vi "Read Shake Data.vi"(8 "error in (no error)":errorcluster, 11 "Abstract Shake Monitor in":refnum<class "Abstract Shake Monitor.lvclass">) -> (0 "error out":errorcluster, 1 "Shake Amplitude (g)":dbl, 2 "Shake Frequency (Hz)":dbl, 3 "Abstract Shake Monitor out":refnum<class "Abstract Shake Monitor.lvclass">)   [LabVIEW 2020, in "Shaker Controller.lvlib" / "Abstract Shake Monitor.lvclass"]
uses:
  Abstract Shake Monitor.lvclass
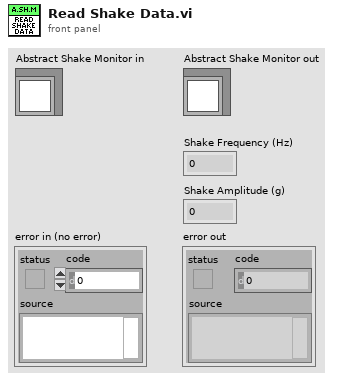
[diagram p1: front panel]
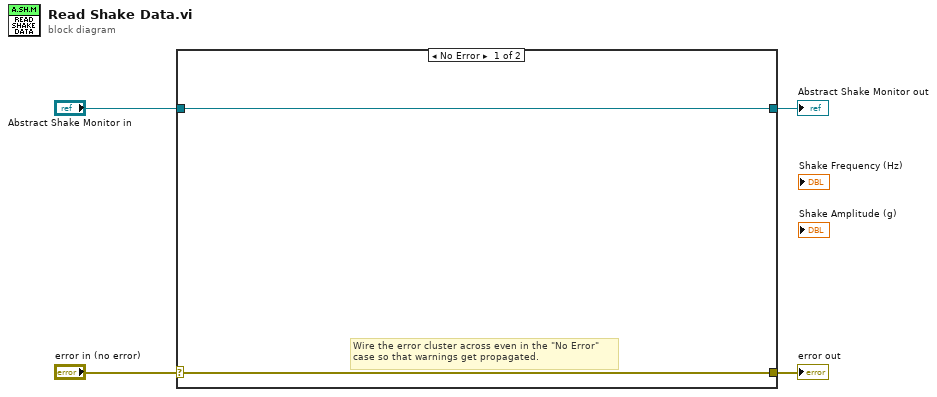
[diagram p0: block diagram]
diagram:
  n1 = case shown="No Error" "error in (no error)" {
    selector: "error in (no error)" -> [w5 w8]
    tunnel: [w5 w8] -> w3
    tunnel: [w6 w7] -> w1
    tunnel: "Abstract Shake Monitor in" -> [w6 w7]
    frame No Error {
      # "Wire the error cluster across even in the \"No Error\"\ncase so that warnings get propagated."
    }
    frame Error {
    }
  }
  "error out" <- w3
  "Abstract Shake Monitor out" <- w1
